vi "shut down sequence.vi"(11 "queues":T1) -> ()   [LabVIEW 2018]
uses:
  type defs/Queues.ctl
  supporting VIs/polymorphic VIs/enqueue for message handler.vi
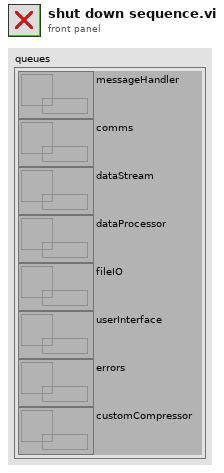
[diagram p1: front panel]
types:
  T1 = typedef "Queues.ctl" = cluster{"messageHandler":refnum<queue>, "comms":refnum<queue>, "dataStream":refnum<queue>, "dataProcessor":refnum<queue>, "fileIO":refnum<queue>, "userInterface":refnum<queue>, "errors":refnum<queue>, "customCompressor":refnum<queue>}
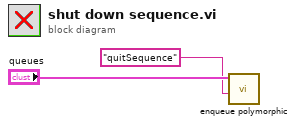
[diagram p0: block diagram]
diagram:
  n1 = call-poly "enqueue polymorphic.vi"("message"="quitSequence", "Queues"="queues") -> ()  [unwired: 9 in, 1 out]
